vi "Variant with Type Information to Strings.vi"(8 "error in (no error)":errorcluster, 11 "Variant":variant) -> (0 "error out":errorcluster, 2 "Data":string, 3 "Datatype":string)   [LabVIEW 2020, in "LUnit Test Vector.lvclass"]
uses:
  LUnit Test Vector.lvclass
  <vilib>/ErrorRing/Error Ring.xnode
  <vilib>/Utility/error.llb/Error Cluster From Error Code.vi
  <vilib>/Utility/Data Type/NI_Data Type.lvlib
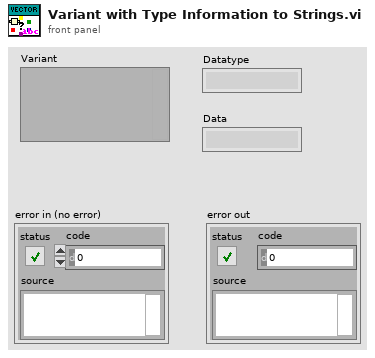
[diagram p1: front panel]
types:
  T1 = typedef "NI_Data Type.lvlib/Data Type.ctl" = enum8{"Invalid Type", "Void", "I8", "I16", "I32", "I64", "U8", "U16", "U32", "U64", "Single Float", "Double Float", "Extended Float", "Single Complex", "Double Complex", "Extended Complex", "Enum U8", "Enum U16", "Enum U32", "Enum U64", "Single Float With Unit", "Double Float With Unit", "Extended Float With Unit", "Single Complex with Unit", "Double Complex with Unit", "Extended Complex with Unit", "Boolean", "String", "Path", "Picture", "Tag", "Array", "Cluster", "Variant", "LV Variant", "Waveform", "Timestamp", "Digital Waveform", "Digital Data", "ExpressData", "Refnum", "External Data", "VI", "Poly VI", "LabVIEW Class Instance", "Fixed Point", "Set Collection", "Map Collection"}
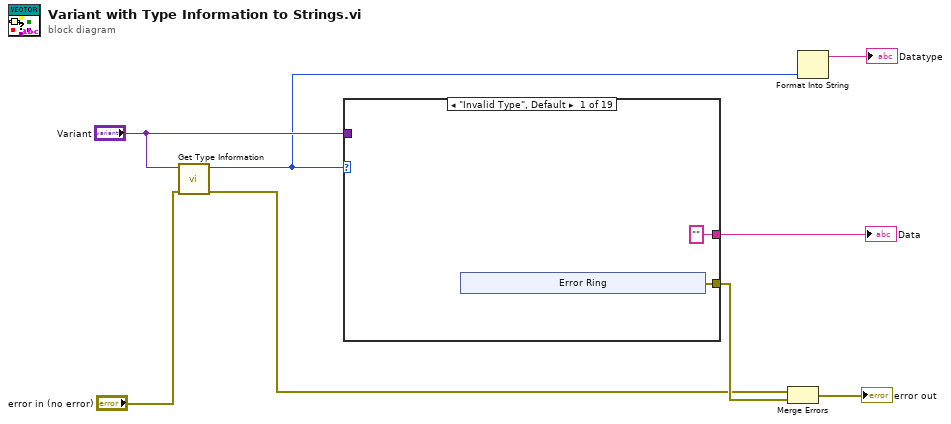
[diagram p0: block diagram]
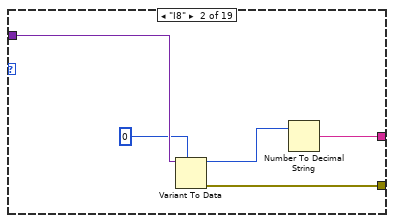
[diagram p2: hidden frame]
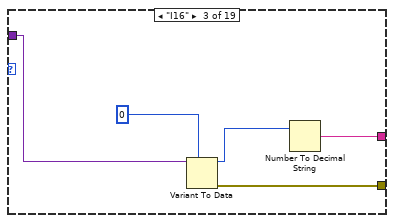
[diagram p3: hidden frame]
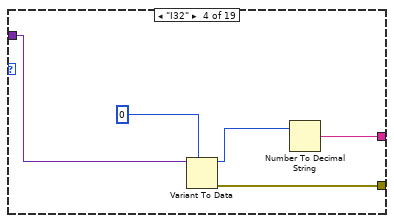
[diagram p4: hidden frame]
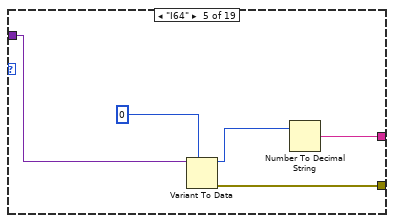
[diagram p5: hidden frame]
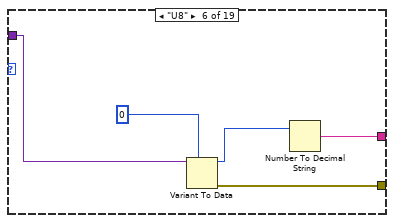
[diagram p6: hidden frame]
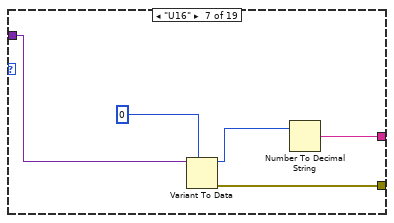
[diagram p7: hidden frame]
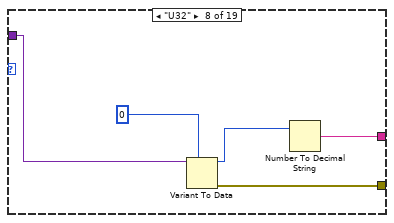
[diagram p8: hidden frame]
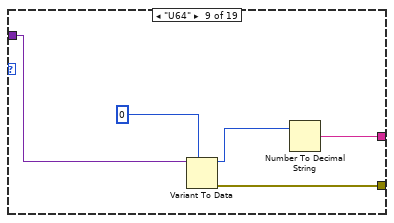
[diagram p9: hidden frame]
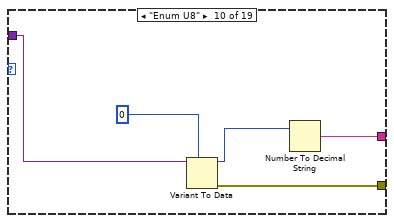
[diagram p10: hidden frame]
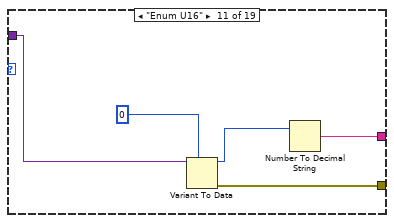
[diagram p11: hidden frame]
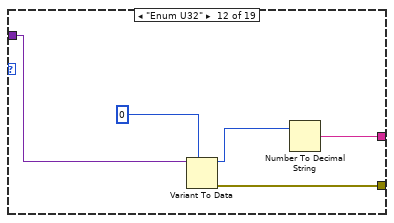
[diagram p12: hidden frame]
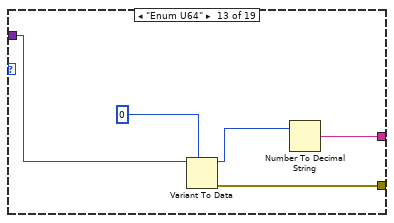
[diagram p13: hidden frame]
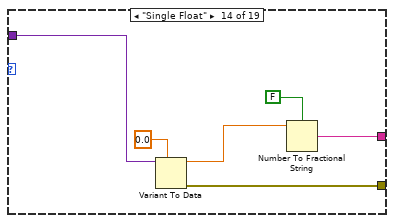
[diagram p14: hidden frame]
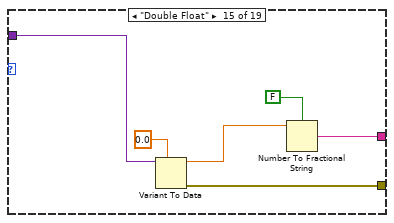
[diagram p15: hidden frame]
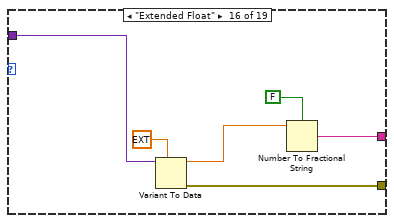
[diagram p16: hidden frame]
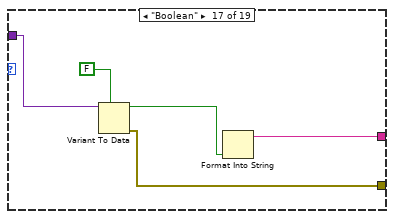
[diagram p17: hidden frame]
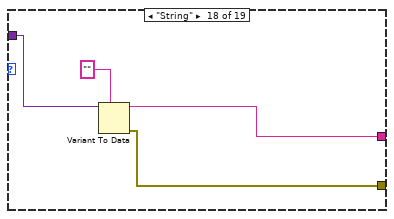
[diagram p18: hidden frame]
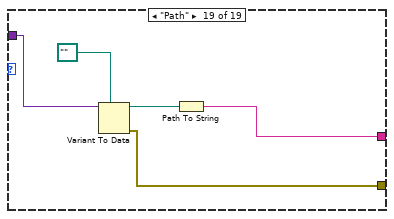
[diagram p19: hidden frame]
diagram:
  n1 = call <vilib>:"Get Type Information.vi"("error in (no error)"="error in (no error)", "variant"="Variant") -> ("error out"=w5:errorcluster, "type"=w2:T1)  [unwired: 5 in, 3 out]
  n2 = case shown="\"Invalid Type\", Default" w2 {
    tunnel: [w10 w17 w22 w27 w32 w37 w42 w47 w52 w57 w62 w67 w72 w78 w84 w90 w93 w98 w104] -> w8
    tunnel: "Variant" -> [_ w19 w23 w28 w33 w38 w43 w48 w53 w58 w63 w68 w73 w79 w85 w91 w96 w100 w106]
    tunnel: ["" w15 w20 w25 w30 w35 w40 w45 w50 w55 w60 w65 w70 w75 w81 w87 w94 w99 w102] -> w3
    frame "Invalid Type", Default {
      n3 = xnode "Error Ring"() -> ("error out"=w10:errorcluster)
    }
    frame "I8" {
      n4 = Variant To Data(type=i8 0 ("default (0 I32)"), Variant=w19) -> (data=w16:i8, error out=w17:errorcluster)  [unwired: 1 in]
      n5 = Number To Decimal String(number=w16) -> (decimal integer string=w15:string)  [unwired: 1 in]
    }
    frame "I16" {
      n6 = Variant To Data(type=i16 0 ("default (0 I32)"), Variant=w23) -> (data=w21:i16, error out=w22:errorcluster)  [unwired: 1 in]
      n7 = Number To Decimal String(number=w21) -> (decimal integer string=w20:string)  [unwired: 1 in]
    }
    frame "I32" {
      n8 = Variant To Data(type=0 ("default (0 I32)"), Variant=w28) -> (data=w26:i32, error out=w27:errorcluster)  [unwired: 1 in]
      n9 = Number To Decimal String(number=w26) -> (decimal integer string=w25:string)  [unwired: 1 in]
    }
    frame "I64" {
      n10 = Variant To Data(type=i64 0 ("default (0 I32)"), Variant=w33) -> (data=w31:i64, error out=w32:errorcluster)  [unwired: 1 in]
      n11 = Number To Decimal String(number=w31) -> (decimal integer string=w30:string)  [unwired: 1 in]
    }
    frame "U8" {
      n12 = Variant To Data(type=u8 0 ("default (0 I32)"), Variant=w38) -> (data=w36:u8, error out=w37:errorcluster)  [unwired: 1 in]
      n13 = Number To Decimal String(number=w36) -> (decimal integer string=w35:string)  [unwired: 1 in]
    }
    frame "U16" {
      n14 = Variant To Data(type=u16 0 ("default (0 I32)"), Variant=w43) -> (data=w41:u16, error out=w42:errorcluster)  [unwired: 1 in]
      n15 = Number To Decimal String(number=w41) -> (decimal integer string=w40:string)  [unwired: 1 in]
    }
    frame "U32" {
      n16 = Variant To Data(type=u32 0 ("default (0 I32)"), Variant=w48) -> (data=w46:u32, error out=w47:errorcluster)  [unwired: 1 in]
      n17 = Number To Decimal String(number=w46) -> (decimal integer string=w45:string)  [unwired: 1 in]
    }
    frame "U64" {
      n18 = Variant To Data(type=u64 0 ("default (0 I32)"), Variant=w53) -> (data=w51:u64, error out=w52:errorcluster)  [unwired: 1 in]
      n19 = Number To Decimal String(number=w51) -> (decimal integer string=w50:string)  [unwired: 1 in]
    }
    frame "Enum U8" {
      n20 = Variant To Data(type=u8 0 ("default (0 I32)"), Variant=w58) -> (data=w56:u8, error out=w57:errorcluster)  [unwired: 1 in]
      n21 = Number To Decimal String(number=w56) -> (decimal integer string=w55:string)  [unwired: 1 in]
    }
    frame "Enum U16" {
      n22 = Variant To Data(type=u16 0 ("default (0 I32)"), Variant=w63) -> (data=w61:u16, error out=w62:errorcluster)  [unwired: 1 in]
      n23 = Number To Decimal String(number=w61) -> (decimal integer string=w60:string)  [unwired: 1 in]
    }
    frame "Enum U32" {
      n24 = Variant To Data(type=u32 0 ("default (0 I32)"), Variant=w68) -> (data=w66:u32, error out=w67:errorcluster)  [unwired: 1 in]
      n25 = Number To Decimal String(number=w66) -> (decimal integer string=w65:string)  [unwired: 1 in]
    }
    frame "Enum U64" {
      n26 = Variant To Data(type=u64 0 ("default (0 I32)"), Variant=w73) -> (data=w71:u64, error out=w72:errorcluster)  [unwired: 1 in]
      n27 = Number To Decimal String(number=w71) -> (decimal integer string=w70:string)  [unwired: 1 in]
    }
    frame "Single Float" {
      n28 = Variant To Data(type=sgl 0.0, Variant=w79) -> (data=w76:sgl, error out=w78:errorcluster)  [unwired: 1 in]
      n29 = Number To Fractional String(use system decimal point (T)=FALSE, number=w76) -> (F-format string=w75:string)  [unwired: 2 in]
    }
    frame "Double Float" {
      n30 = Variant To Data(type=0.0, Variant=w85) -> (data=w82:dbl, error out=w84:errorcluster)  [unwired: 1 in]
      n31 = Number To Fractional String(use system decimal point (T)=FALSE, number=w82) -> (F-format string=w81:string)  [unwired: 2 in]
    }
    frame "Extended Float" {
      n32 = Variant To Data(type=ext 0.0, Variant=w91) -> (data=w88:ext, error out=w90:errorcluster)  [unwired: 1 in]
      n33 = Number To Fractional String(use system decimal point (T)=FALSE, number=w88) -> (F-format string=w87:string)  [unwired: 2 in]
    }
    frame "Boolean" {
      n34 = Variant To Data(type=FALSE, Variant=w96) -> (data=w95:bool, error out=w93:errorcluster)  [unwired: 1 in]
      n35 = Format Into String(w95) -> (resulting string=w94:string)  [unwired: 3 in, 1 out]
    }
    frame "String" {
      n36 = Variant To Data(type="", Variant=w100) -> (data=w99:string, error out=w98:errorcluster)  [unwired: 1 in]
    }
    frame "Path" {
      n37 = Variant To Data(type=path "" ("path"), Variant=w106) -> (data=w105:path, error out=w104:errorcluster)  [unwired: 1 in]
      n38 = Path To String(path=w105) -> (string=w102:string)
    }
  }
  "Data" <- w3
  n39 = Merge Errors(w5, w8) -> (→"error out":errorcluster)
  n40 = Format Into String(w2) -> (resulting string=→"Datatype":string)  [unwired: 3 in, 1 out]
